vi "OSA_example_traces.vi"() -> ()   [LabVIEW 2010]
doc: "A trace contain data arrays and properties for a spectrum or an interferogram allocated and handled by FTSLib.dll, (see spectrum_t). \n\nThe OSA200 labview driver allocates 10 spectrum traces and 2 interferogram ditto per default, with the same array sizes as the labview allocated arrays in buffer.vi, (see the init.vi buffer size and traces input parameters). \n\nTrace data can be created either from an acquisition, (see the acquisition vis), file IO read or as a result from trace calculations, (trace math).\n\nThe traces functions are useful when several spectra/interferograms are required, (the labview buffer supports only one spectrum/interferogram), and for data transfer to the OSA200 application GUI, (file IO). \n\nTrace properties, such as name and comment strings, can be edited.\n\nUse trace_toLVBuffer.vi and buffer_get.vi to access trace data from within Labview. Trace data, (which resides in FTSLib.dll memory space), must be transferred to Labview memory space in order to handle trace interferogram and spectrum data with Labview operators and functions."
uses:
  _misc/Thorlabs_FTS_misc.llb/graph_spectrum.ctl
  _misc/Thorlabs_FTS_misc.llb/graph_interferogram.ctl
  _OSA_class/misc_examples/action_trace.ctl
  _misc/Thorlabs_FTS_misc.llb/OSA_virtualModel.ctl
  _misc/Thorlabs_FTS_misc.llb/OSA_virtualSource_RS.ctl
  _OSA_class/typeDef/acq_dataType.ctl
  _OSA_class/OSA.lvclass
  OSA20X_misc.lvlib
panel:
  in  "saveToFile multiple butt":bool
  in  "readFromFile multiple butt":bool
  in  "file format (SPF2)":T1(ring)=enum."SPF2"
  in  "trace set comment":string
  in  "exit butt":bool
  in  "Tab Control":enum32{"interferogram", "spectrum"}(tab)=enum."spectrum"
  out "Intensity Graph Interferogram":T2
  in  "trace interferogram":i32[](listbox)
  in  "trace spectrum":i32[](listbox)
  out "Intensity Graph spectrum":T3
  in  "readFromFile butt":bool
  in  "saveToFile butt":bool
  in  "acquire butt":bool
  in  "display butt":bool
  in  "trace set name":string
  in  "virtual OSA":bool=TRUE
  # "hold ctrl key"
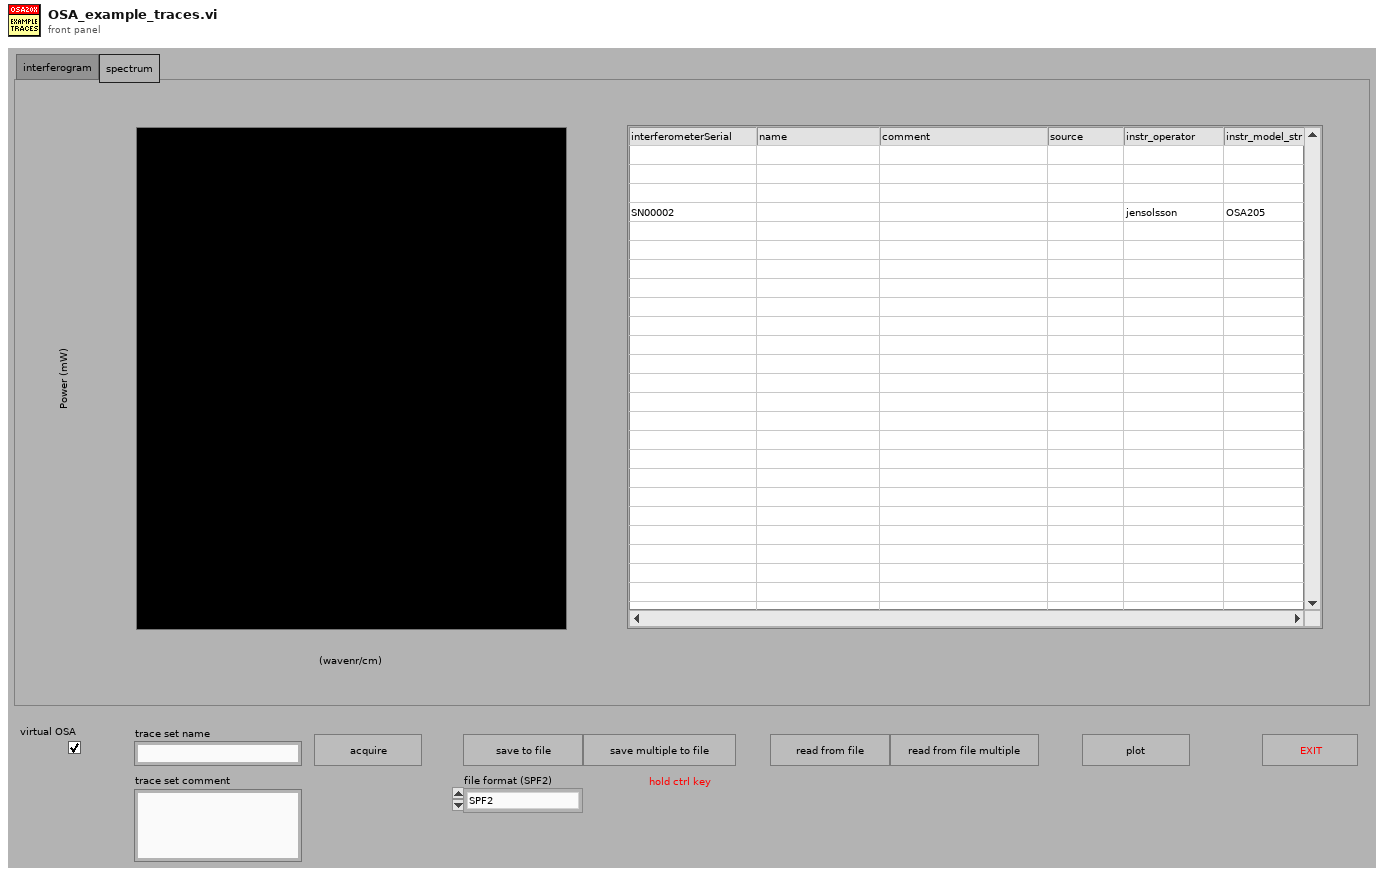
[diagram p1: front panel]
types:
  T1 = enum16{"SPC", "CSV", "SPF2", "TXT", "MAT_V5", "CSV_ZIP", "TXT_ZIP", "JCAMPDX"}
  T2 = typedef "OSA20X_misc.lvlib/graph_interferogram.ctl" = i32[][]
  T3 = typedef "OSA20X_misc.lvlib/graph_spectrum.ctl" = i32[][]
  T4 = typedef "OSA20X_misc.lvlib/OSA_virtualSource_RS.ctl" = enum16{"VIRTUAL_REDSTONE_SOURCE_UNKNOWN", "VIRTUAL_REDSTONE_SOURCE_LLD_DFB_1530", "VIRTUAL_REDSTONE_SOURCE_SLD_1550nm", "VIRTUAL_REDSTONE_SOURCE_LASER_4600nm", "VIRTUAL_REDSTONE_SOURCE_BLACKBODY1500K", "VIRTUAL_REDSTONE_SOURCE_BLACKBODY1500K_H2O"}
  T5 = cluster{"OSA200":cluster{"waveCenter (nm)":dbl, "FWHM (nm)":dbl, "peakAmplitude":dbl}, "OSA300":T4}
  T6 = typedef "OSA20X_misc.lvlib/OSA_virtualModel.ctl" = enum16{"OSA201", "OSA201C", "OSA202", "OSA202C", "OSA203", "OSA203B", "OSA203C", "OSA205", "OSA205C", "REDSTONE301", "REDSTONE305"}
  T7 = cluster{"nr interferogram (2)":i32, "nr spectrum (10)":i32}
  T8 = typedef "OSA.lvclass/action_trace.ctl" = enum16{"init", "acquisition", "getTrace_info", "displayTrace", "sourceSelect_virtual", "file_IO_write", "file_IO_write_multiple", "file_IO_read", "file_IO_read_multiple", "user", "exit"}
  T9 = cluster{"trace spectrum":refnum<vi>, "trace interferogram":refnum<vi>, "Tab Control":refnum<vi>}
  T10 = typedef "OSA.lvclass/acq_dataType.ctl" = enum16{"none", "interferogram", "spectrum"}
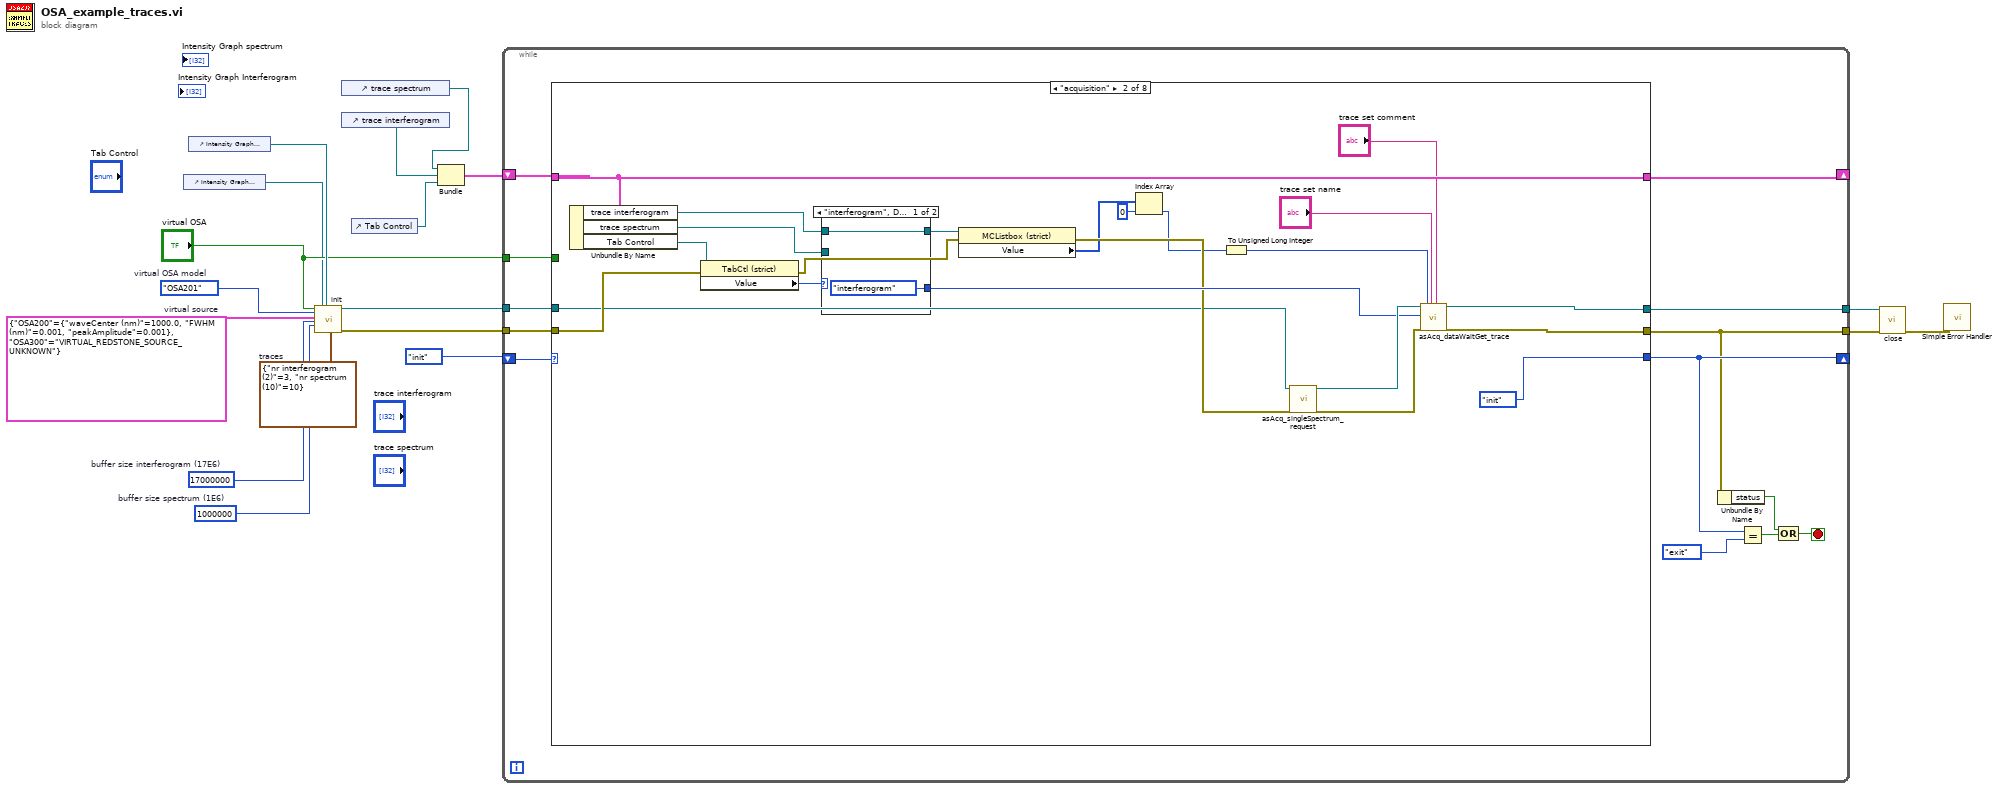
[diagram p0: block diagram]
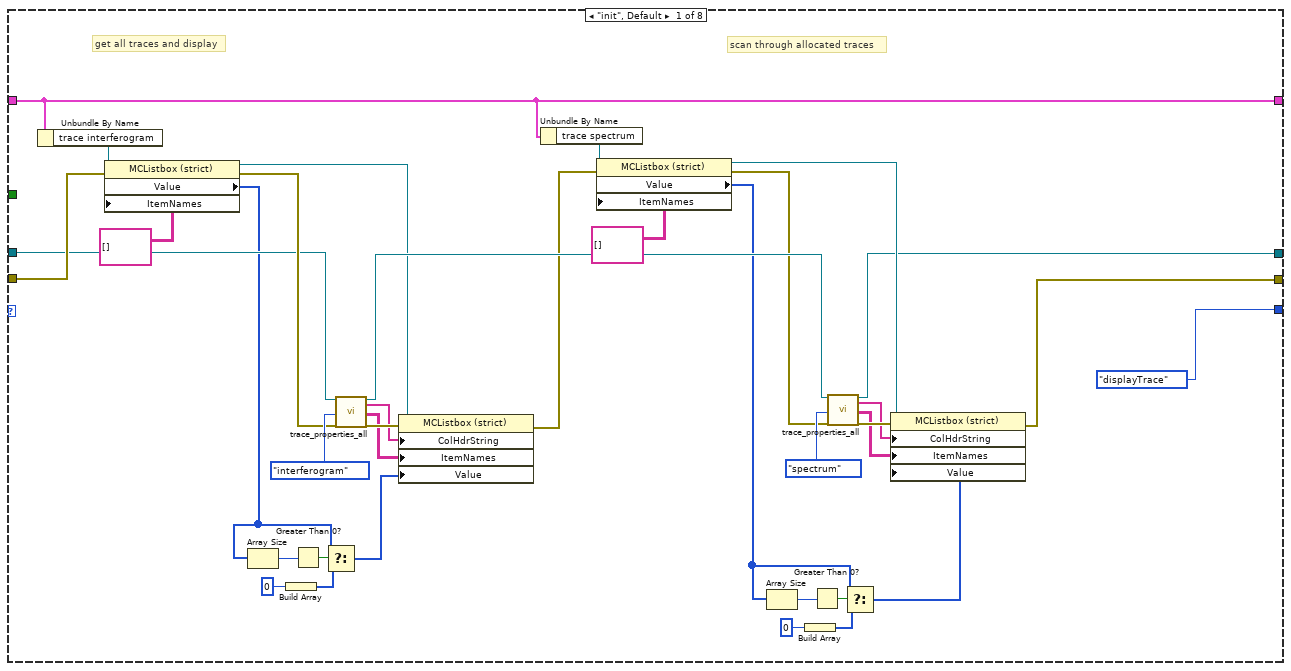
[diagram p2: hidden frame]
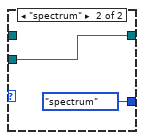
[diagram p3: hidden frame]
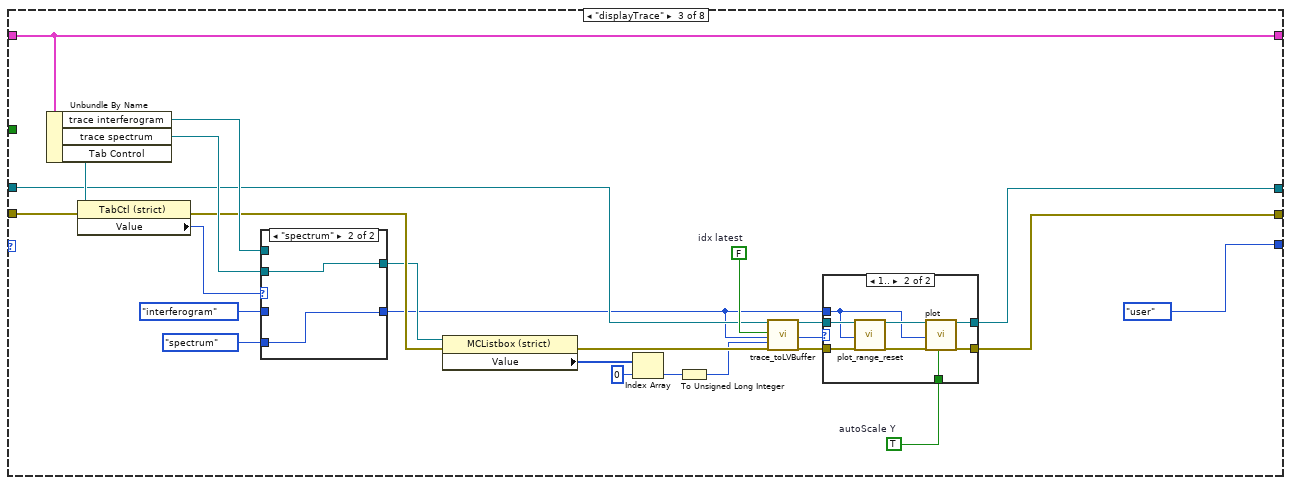
[diagram p4: hidden frame]
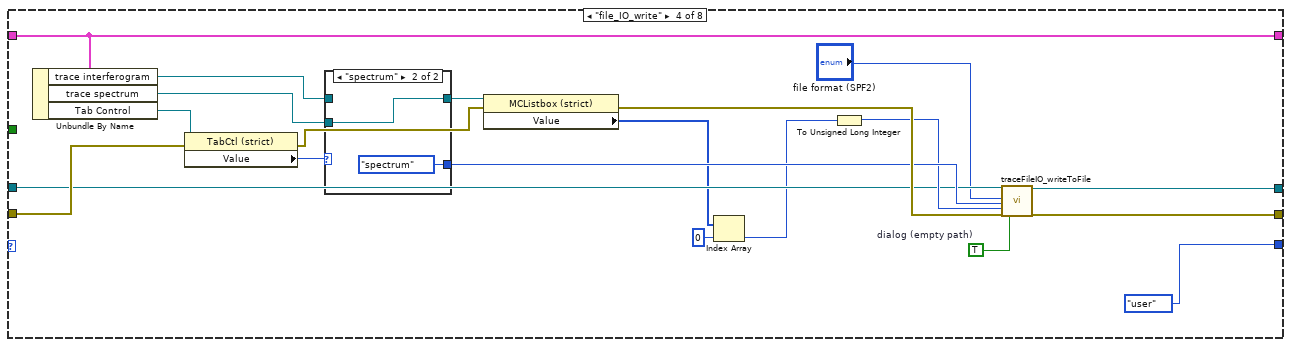
[diagram p7: hidden frame]
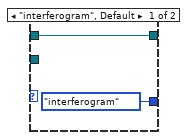
[diagram p8: hidden frame]
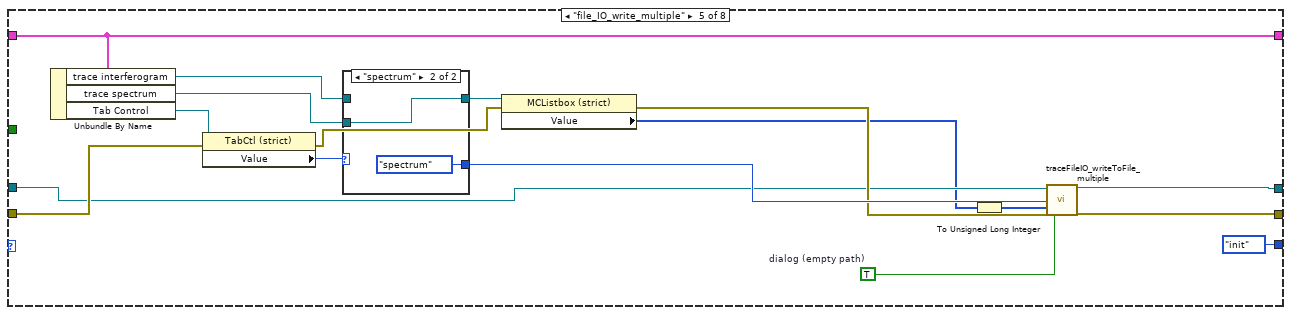
[diagram p9: hidden frame]
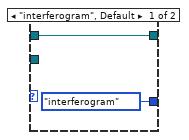
[diagram p10: hidden frame]
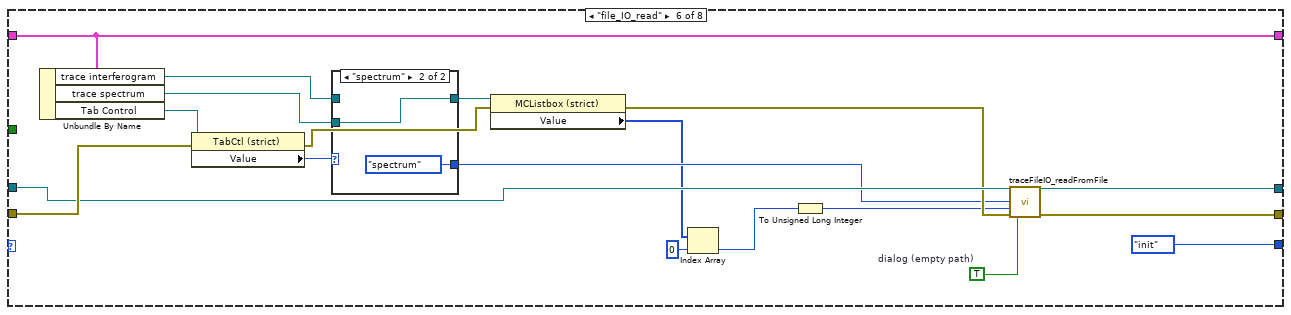
[diagram p11: hidden frame]
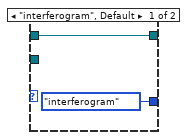
[diagram p12: hidden frame]
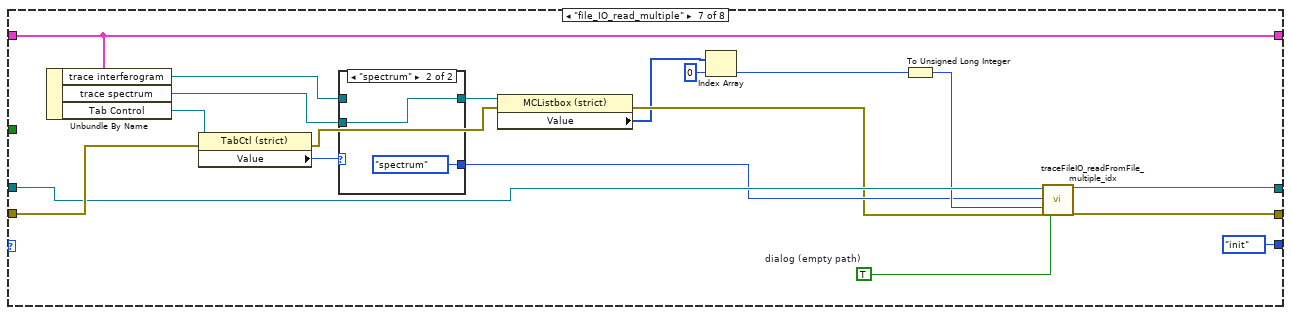
[diagram p13: hidden frame]
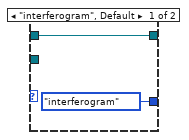
[diagram p14: hidden frame]
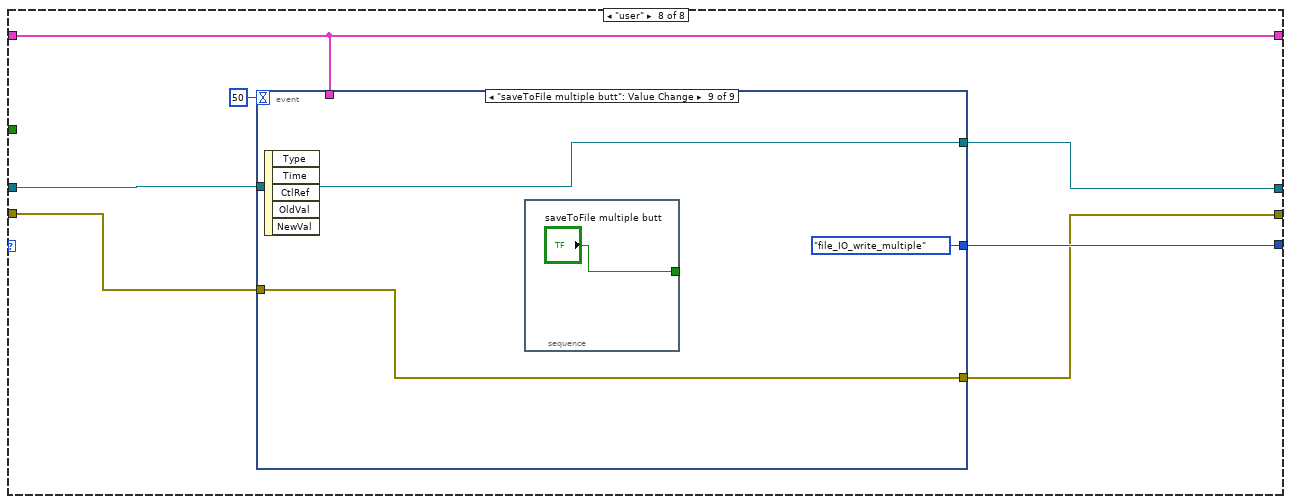
[diagram p15: hidden frame]
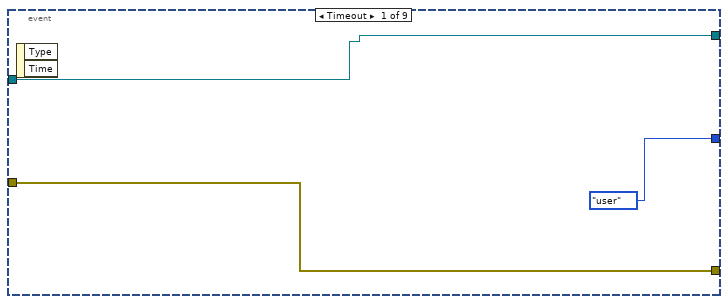
[diagram p16: hidden frame]
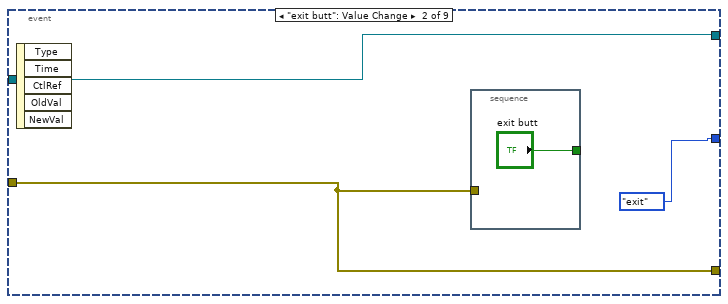
[diagram p17: hidden frame]
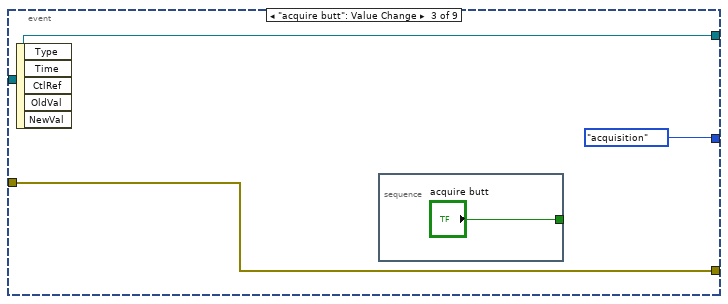
[diagram p18: hidden frame]
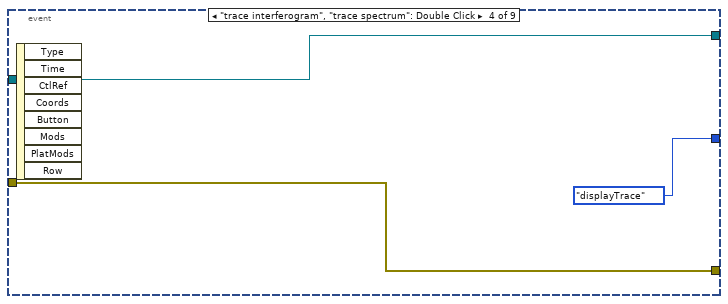
[diagram p19: hidden frame]
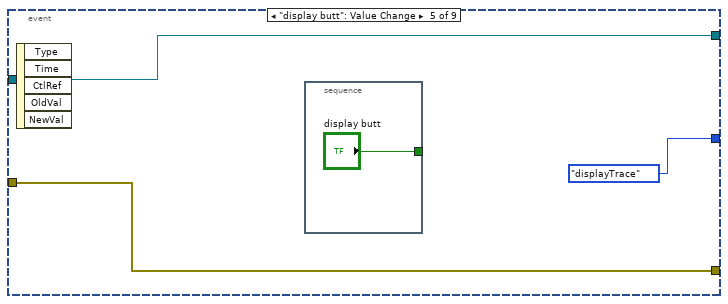
[diagram p20: hidden frame]
diagram:
  w1 = T5 {"OSA200"={"waveCenter (nm)"=1000.0, "FWHM (nm)"=0.001, "peakAmplitude"=0.001}, "OSA300"=enum."VIRTUAL_REDSTONE_SOURCE_UNKNOWN"}  # virtual source
  w2 = OSA_virtualModel."OSA201"  # virtual OSA model
  w3 = 1000000  # buffer size spectrum (1E6)
  w4 = 17000000  # buffer size interferogram (17E6)
  w5 = T7 {"nr interferogram (2)"=3, "nr spectrum (10)"=10}  # traces
  n1 = control-ref of="Intensity Graph Interferogram"() -> (w15:refnum<vi>)
  n2 = control-ref of="Intensity Graph spectrum"() -> (w18:refnum<vi>)
  n3 = call "init.vi"("virtual OSA"="virtual OSA", "virtual OSA model"=w2, "virtual source"=w1, "buffer size interferogram (17E6)"=w4, "buffer size spectrum (1E6)"=w3, "Graph Intrfrgrm"=w15, "Graph Spectrum"=w18, "traces"=w5) -> ("duplicate reference"=w8:refnum<class "OSA.lvclass">, "error out"=w17:errorcluster)  [unwired: 7 in, 3 out]
  n4 = control-ref of="trace spectrum"() -> (w12:refnum<vi>)
  n5 = control-ref of="trace interferogram"() -> (w11:refnum<vi>)
  n6 = control-ref of="Tab Control"() -> (w9:refnum<vi>)
  n7 = Bundle("trace spectrum"=w12, "trace interferogram"=w11, "Tab Control"=w9) -> (w10:T9)  [unwired: 1 in]
  n8 = while {
    shift-right: [w26] -> _
    shift-left: action_trace."init" ("Enum") -> [w31]
    tunnel: w17 -> [w29]
    tunnel: "virtual OSA" -> [w30]
    tunnel: [w24] -> w14
    shift-right: [w27] -> _
    shift-left: w10 -> [w28]
    tunnel: w8 -> [w21]
    tunnel: [w20] -> w7
    stop <- w22 stop-if-true
    n9 = case shown="\"acquisition\"" w31 {
      tunnel: w30 -> [_ _ _ _ _ _ _ _]
      tunnel: [action_trace."displayTrace" ("Enum") action_trace."init" ("Enum") action_trace."user" ("Enum") action_trace."user" ("Enum") action_trace."init" ("Enum") action_trace."init" ("Enum") action_trace."init" ("Enum") w230] -> w26
      tunnel: w29 -> [w63 w84 w118 w146 w163 w190 w213 w227]
      tunnel: w28 -> [w54 w85 w116 w140 w164 w189 w212 w228]
      tunnel: [w49 w86 w95 w144 w160 w186 w209 w226] -> w24
      tunnel: [w54 w85 w116 w140 w164 w189 w212 w228] -> w27
      tunnel: w21 -> [w45 w72 w101 w138 w162 w187 w211 w225]
      tunnel: [w46 w73 w94 w139 w161 w188 w210 w224] -> w20
      frame "init", Default {
        # "scan through allocated traces"
        # "get all traces and display"
        n10 = Unbundle By Name(w54) -> ("trace interferogram"=w62:refnum<vi>)
        n11 = property class="MCListbox (strict)"(reference=w62, error in=w63, "ItemNames"=string[][] [] ("Item Names")) -> (reference out=w48:refnum<vi>, error out=w53:errorcluster, "Value"=w33:i32[])
        n12 = Array Size(array=w33) -> (size(s)=w36:i32)
        n13 = Build Array(0 ("f")) -> (w34:i32[])
        n14 = Greater Than 0?(x=w36) -> (x > 0?=w37:bool)
        n15 = Select(t=w33, s=w37, f=w34) -> (s? t:f=w32:i32[])
        n16 = call "trace_properties_all.vi"("reference in"=w45, "dataType"=acq_dataType."interferogram", "error in (no error)"=w53) -> ("reference out"=w52:refnum<class "OSA.lvclass">, "properties"=w65:string[], "property values"=w64:string[][], "error out"=w66:errorcluster)  [unwired: 13 in]
        n17 = property class="MCListbox (strict)"(reference=w48, error in=w66, "ColHdrString"=w65, "ItemNames"=w64, "Value"=w32) -> (error out=w51:errorcluster)  [unwired: 1 out]
        n18 = Unbundle By Name(w54) -> ("trace spectrum"=w56:refnum<vi>)
        n19 = property class="MCListbox (strict)"(reference=w56, error in=w51, "ItemNames"=string[][] [] ("Item Names")) -> (reference out=w47:refnum<vi>, error out=w50:errorcluster, "Value"=w42:i32[])
        n20 = Array Size(array=w42) -> (size(s)=w40:i32)
        n21 = Build Array(0 ("f")) -> (w38:i32[])
        n22 = Greater Than 0?(x=w40) -> (x > 0?=w43:bool)
        n23 = call "trace_properties_all.vi"("reference in"=w52, "dataType"=acq_dataType."spectrum", "error in (no error)"=w50) -> ("reference out"=w46:refnum<class "OSA.lvclass">, "properties"=w58:string[], "property values"=w57:string[][], "error out"=w59:errorcluster)  [unwired: 13 in]
        n24 = Select(t=w42, s=w43, f=w38) -> (s? t:f=w41:i32[])
        n25 = property class="MCListbox (strict)"(reference=w47, error in=w59, "ColHdrString"=w58, "ItemNames"=w57, "Value"=w41) -> (error out=w49:errorcluster)  [unwired: 1 out]
      }
      frame "acquisition" {
        n26 = Unbundle By Name(w85) -> ("trace interferogram"=w80:refnum<vi>, "trace spectrum"=w81:refnum<vi>, "Tab Control"=w83:refnum<vi>)
        n27 = property class="TabCtl (strict)"(reference=w83, error in=w84) -> (error out=w77:errorcluster, "Value"=w82:enum32{"interferogram", "spectrum"})  [unwired: 1 out]
        n28 = case shown="\"interferogram\", Default" w82 {
          tunnel: w81 -> [_ w93]
          tunnel: w80 -> [w90 _]
          tunnel: [acq_dataType."interferogram" ("dataType") acq_dataType."spectrum" ("dataType")] -> w79
          tunnel: [w90 w93] -> w78
          frame "interferogram", Default {
          }
          frame "spectrum" {
          }
        }
        n29 = property class="MCListbox (strict)"(reference=w78, error in=w77) -> (error out=w75:errorcluster, "Value"=w69:i32[])  [unwired: 1 out]
        n30 = Index Array(array=w69, index=0) -> (element=w68:i32)
        n31 = To Unsigned Long Integer(number=w68) -> (unsigned 32bit integer=w87:u32)
        n32 = call "asAcq_singleSpectrum_request.vi"("reference"=w72, "error in (no error)"=w75) -> ("duplicate reference"=w88:refnum<class "OSA.lvclass">, "error out"=w89:errorcluster)  [unwired: 16 in]
        n33 = call "asAcq_dataWaitGet_trace.vi"("reference"=w88, "dataType"=w79, "error in (no error)"=w89, "trace index"=w87, "trace set name"="trace set name", "trace set comment"="trace set comment") -> ("duplicate reference"=w73:refnum<class "OSA.lvclass">, "error out"=w86:errorcluster)  [unwired: 10 in, 2 out]
      }
      frame "displayTrace" {
        w102 = FALSE  # idx latest
        w96 = TRUE  # autoScale Y
        n34 = Unbundle By Name(w116) -> ("trace interferogram"=w112:refnum<vi>, "trace spectrum"=w113:refnum<vi>, "Tab Control"=w117:refnum<vi>)
        n35 = property class="TabCtl (strict)"(reference=w117, error in=w118) -> (error out=w104:errorcluster, "Value"=w114:enum32{"interferogram", "spectrum"})  [unwired: 1 out]
        n36 = case shown="\"spectrum\"" w114 {
          tunnel: w113 -> [_ w131]
          tunnel: w112 -> [w130 _]
          tunnel: acq_dataType."interferogram" ("dataType") -> [w129 _]
          tunnel: acq_dataType."spectrum" ("dataType") -> [_ w132]
          tunnel: [w129 w132] -> w98
          tunnel: [w130 w131] -> w103
          frame "interferogram", Default {
          }
          frame "spectrum" {
          }
        }
        n37 = property class="MCListbox (strict)"(reference=w103, error in=w104) -> (error out=w106:errorcluster, "Value"=w108:i32[])  [unwired: 1 out]
        n38 = Index Array(array=w108, index=0) -> (element=w107:i32)
        n39 = To Unsigned Long Integer(number=w107) -> (unsigned 32bit integer=w105:u32)
        n40 = call "trace_toLVBuffer.vi"("reference in"=w101, "idx latest"=w102, "dataType"=w98, "trace idx"=w105, "error in (no error)"=w106) -> ("reference out"=w100:refnum<class "OSA.lvclass">, "trace length"=w97:u32, "error out"=w99:errorcluster)  [unwired: 12 in]
        n41 = case shown="1.." w97 {
          tunnel: w100 -> [w119 w128]
          tunnel: w99 -> [w120 w127]
          tunnel: w98 -> [_ w124]
          tunnel: [w119 w123] -> w94
          tunnel: [w120 w122] -> w95
          tunnel: w96 -> [_ w121]
          frame 0, Default {
          }
          frame 1.. {
            n42 = call "plot_range_reset.vi"("reference"=w128, "dataType"=w124, "error in (no error)"=w127) -> ("duplicate reference"=w125:refnum<class "OSA.lvclass">, "error out"=w126:errorcluster)  [unwired: 15 in]
            n43 = call "plot.vi"("reference"=w125, "dataType"=w124, "error in (no error)"=w126, "autoScale Y"=w121) -> ("duplicate reference"=w123:refnum<class "OSA.lvclass">, "error out"=w122:errorcluster)  [unwired: 14 in]
          }
        }
      }
      frame "file_IO_write" {
        w143 = TRUE  # dialog (empty path)
        n44 = Unbundle By Name(w140) -> ("trace interferogram"=w149:refnum<vi>, "trace spectrum"=w150:refnum<vi>, "Tab Control"=w152:refnum<vi>)
        n45 = property class="TabCtl (strict)"(reference=w152, error in=w146) -> (error out=w147:errorcluster, "Value"=w151:enum32{"interferogram", "spectrum"})  [unwired: 1 out]
        n46 = case shown="\"spectrum\"" w151 {
          tunnel: w150 -> [_ w156]
          tunnel: w149 -> [w153 _]
          tunnel: [acq_dataType."interferogram" ("dataType") acq_dataType."spectrum" ("dataType")] -> w142
          tunnel: [w153 w156] -> w148
          frame "interferogram", Default {
          }
          frame "spectrum" {
          }
        }
        n47 = property class="MCListbox (strict)"(reference=w148, error in=w147) -> (error out=w145:errorcluster, "Value"=w134:i32[])  [unwired: 1 out]
        n48 = Index Array(array=w134, index=0) -> (element=w133:i32)
        n49 = To Unsigned Long Integer(number=w133) -> (unsigned 32bit integer=w141:u32)
        n50 = call "traceFileIO_writeToFile.vi"("reference in"=w138, "file format (SPF2)"="file format (SPF2)", "dataType"=w142, "trace idx"=w141, "error in (no error)"=w145, "dialog (empty path)"=w143) -> ("reference out"=w139:refnum<class "OSA.lvclass">, "error out"=w144:errorcluster)  [unwired: 9 in, 3 out]
      }
      frame "file_IO_write_multiple" {
        w167 = TRUE  # dialog (empty path)
        n51 = Unbundle By Name(w164) -> ("trace interferogram"=w170:refnum<vi>, "trace spectrum"=w171:refnum<vi>, "Tab Control"=w173:refnum<vi>)
        n52 = property class="TabCtl (strict)"(reference=w173, error in=w163) -> (error out=w168:errorcluster, "Value"=w172:enum32{"interferogram", "spectrum"})  [unwired: 1 out]
        n53 = case shown="\"spectrum\"" w172 {
          tunnel: w171 -> [_ w177]
          tunnel: w170 -> [w174 _]
          tunnel: [acq_dataType."interferogram" ("dataType") acq_dataType."spectrum" ("dataType")] -> w166
          tunnel: [w174 w177] -> w169
          frame "interferogram", Default {
          }
          frame "spectrum" {
          }
        }
        n54 = property class="MCListbox (strict)"(reference=w169, error in=w168) -> (error out=w165:errorcluster, "Value"=w159:i32[])  [unwired: 1 out]
        n55 = To Unsigned Long Integer(number=w159) -> (unsigned 32bit integer=w158:u32[])
        n56 = call "traceFileIO_writeToFile_multiple.vi"("reference in"=w162, "dataType"=w166, "traces idx"=w158, "error in (no error)"=w165, "dialog (empty path)"=w167) -> ("reference out"=w161:refnum<class "OSA.lvclass">, "error out"=w160:errorcluster)  [unwired: 10 in, 3 out]
      }
      frame "file_IO_read" {
        w182 = TRUE  # dialog (empty path)
        n57 = Unbundle By Name(w189) -> ("trace interferogram"=w193:refnum<vi>, "trace spectrum"=w194:refnum<vi>, "Tab Control"=w196:refnum<vi>)
        n58 = property class="TabCtl (strict)"(reference=w196, error in=w190) -> (error out=w191:errorcluster, "Value"=w195:enum32{"interferogram", "spectrum"})  [unwired: 1 out]
        n59 = case shown="\"spectrum\"" w195 {
          tunnel: w194 -> [_ w200]
          tunnel: w193 -> [w197 _]
          tunnel: [acq_dataType."interferogram" ("dataType") acq_dataType."spectrum" ("dataType")] -> w184
          tunnel: [w197 w200] -> w192
          frame "interferogram", Default {
          }
          frame "spectrum" {
          }
        }
        n60 = property class="MCListbox (strict)"(reference=w192, error in=w191) -> (error out=w185:errorcluster, "Value"=w179:i32[])  [unwired: 1 out]
        n61 = Index Array(array=w179, index=0) -> (element=w178:i32)
        n62 = To Unsigned Long Integer(number=w178) -> (unsigned 32bit integer=w183:u32)
        n63 = call "traceFileIO_readFromFile.vi"("reference"=w187, "dataType"=w184, "trace idx"=w183, "error in (no error)"=w185, "dialog (empty path)"=w182) -> ("duplicate reference"=w188:refnum<class "OSA.lvclass">, "error out"=w186:errorcluster)  [unwired: 12 in, 1 out]
      }
      frame "file_IO_read_multiple" {
        w208 = TRUE  # dialog (empty path)
        n64 = Unbundle By Name(w212) -> ("trace interferogram"=w216:refnum<vi>, "trace spectrum"=w217:refnum<vi>, "Tab Control"=w219:refnum<vi>)
        n65 = property class="TabCtl (strict)"(reference=w219, error in=w213) -> (error out=w214:errorcluster, "Value"=w218:enum32{"interferogram", "spectrum"})  [unwired: 1 out]
        n66 = case shown="\"spectrum\"" w218 {
          tunnel: w217 -> [_ w223]
          tunnel: w216 -> [w220 _]
          tunnel: [acq_dataType."interferogram" ("dataType") acq_dataType."spectrum" ("dataType")] -> w206
          tunnel: [w220 w223] -> w215
          frame "interferogram", Default {
          }
          frame "spectrum" {
          }
        }
        n67 = property class="MCListbox (strict)"(reference=w215, error in=w214) -> (error out=w204:errorcluster, "Value"=w202:i32[])  [unwired: 1 out]
        n68 = Index Array(array=w202, index=0) -> (element=w201:i32)
        n69 = To Unsigned Long Integer(number=w201) -> (unsigned 32bit integer=w207:u32)
        n70 = call "traceFileIO_readFromFile_multiple_idx.vi"("reference in"=w211, "dataType"=w206, "trace idx start"=w207, "error in (no error)"=w204, "dialog (empty path)"=w208) -> ("reference out"=w210:refnum<class "OSA.lvclass">, "error out"=w209:errorcluster)  [unwired: 11 in, 2 out]
      }
      frame "user" {
        n71 = event shown="[8] \"saveToFile multiple butt\": Value Change" {
          selector: _ -> [_ _ _ _ _ _ _ _ _]
          dyn-events: _ -> [_ _ _ _ _ _ _ _ _]
          timeout: 50 -> [_ _ _ _ _ _ _ _ _]
          tunnel: [action_trace."user" ("Enum") action_trace."exit" ("Enum") action_trace."acquisition" ("Enum") action_trace."displayTrace" ("Enum") action_trace."displayTrace" ("Enum") action_trace."file_IO_read" ("Enum") action_trace."file_IO_read_multiple" ("Enum") action_trace."file_IO_write" ("Enum") action_trace."file_IO_write_multiple" ("Enum")] -> w230
          tunnel: w228 -> [_ _ _ _ _ _ _ _ _]
          tunnel: w227 -> [w233 w236 w239 w244 w246 w250 w254 w259 w261]
          tunnel: [w233 w236 w239 w244 w246 w250 w254 w259 w261] -> w226
          tunnel: w225 -> [w232 w235 w240 w243 w247 w251 w253 w258 w262]
          tunnel: [w232 w235 w240 w243 w247 w251 w253 w258 w262] -> w224
          event Timeout {
            n72 = event-data() -> ()  [unwired: 1 in, 2 out]
          }
          event "exit butt": Value Change {
            n73 = event-data() -> ()  [unwired: 1 in, 5 out]
            n74 = stacked-sequence {
              tunnel: w236 -> [_]
              tunnel: ["exit butt"] -> _
              frame #0 {
              }
            }
          }
          event "acquire butt": Value Change {
            n75 = event-data() -> ()  [unwired: 1 in, 5 out]
            n76 = stacked-sequence {
              tunnel: ["acquire butt"] -> _
              frame #0 {
              }
            }
          }
          event "trace interferogram", "trace spectrum": Double Click {
            n77 = event-data() -> ()  [unwired: 1 in, 8 out]
          }
          event "display butt": Value Change {
            n78 = event-data() -> ()  [unwired: 1 in, 5 out]
            n79 = stacked-sequence {
              tunnel: ["display butt"] -> _
              frame #0 {
              }
            }
          }
          event "readFromFile butt": Value Change {
            n80 = event-data() -> ()  [unwired: 1 in, 5 out]
            n81 = stacked-sequence {
              tunnel: ["readFromFile butt"] -> _
              frame #0 {
              }
            }
          }
          event "readFromFile multiple butt": Value Change {
            n82 = event-data() -> ()  [unwired: 1 in, 5 out]
            n83 = stacked-sequence {
              tunnel: ["readFromFile multiple butt"] -> _
              frame #0 {
              }
            }
          }
          event "saveToFile butt": Value Change {
            n84 = event-data() -> ()  [unwired: 1 in, 5 out]
            n85 = stacked-sequence {
              tunnel: ["saveToFile butt"] -> _
              frame #0 {
              }
            }
          }
          event "saveToFile multiple butt": Value Change {
            n86 = event-data() -> ()  [unwired: 1 in, 5 out]
            n87 = stacked-sequence {
              tunnel: ["saveToFile multiple butt"] -> _
              frame #0 {
              }
            }
          }
        }
      }
    }
    n88 = Unbundle By Name(w24) -> ("status"=w23:bool)
    n89 = Equal?(x=w26, y=action_trace."exit" ("Enum")) -> (x = y?=w25:bool)
    n90 = Compound Arithmetic op=OR(w23, w25) -> (w22:bool)
  }
  n91 = call "close.vi"("reference"=w7, "error in (no error)"=w14) -> ("error out"=w13:errorcluster)  [unwired: 17 in]
  n92 = call <vilib>:"Simple Error Handler.vi"("error in (no error)"=w13) -> ()  [unwired: 4 in, 5 out]
